vi "Boolean Toggle.vi"(1 "Input":bool) -> (0 "Toggle":bool)   [LabVIEW 2014]
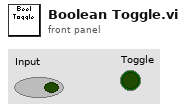
[diagram p1: front panel]
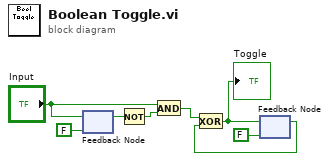
[diagram p0: block diagram]
diagram:
  n1 = feedback-in #1("Input") -> ()
  n2 = feedback #1(FALSE ("Input")) -> (w7:bool)
  n3 = Not(x=w7) -> (.not. x?=w6:bool)
  n4 = And(x="Input", y=w6) -> (x .and. y?=w4:bool)
  n5 = feedback #2(FALSE) -> (w2:bool)
  n6 = Exclusive Or(1:w2, 2:w4) -> (0:w1:bool)
  "Toggle" <- w1
  n7 = feedback-in #2(w1) -> ()
